vi "BoxExecute.vi"(8 "error in (no error)":errorcluster) -> (0 "error out":errorcluster)   [LabVIEW 2023]
uses:
  BoxStatesEnum.ctl
  BoxNoteState.ctl
  <vilib>/Rock Robotics/WPI/ThirdParty/JAS_Junk/TrajLib/TypeDef/PID_ERROR_TOLERANCE.ctl
  <vilib>/Rock Robotics/WPI/ThirdParty/JAS_Junk/TrajLib/VI/BoolCmd_Recv_Internal.vi
  <vilib>/Rock Robotics/WPI/ThirdParty/JAS_Junk/TrajLib/PIDController_AtSetpoint.vi
  <vilib>/Rock Robotics/WPI/ThirdParty/JAS_Junk/TrajLib/PIDController_SetPIDF.vi
  <vilib>/Rock Robotics/WPI/ThirdParty/JAS_Junk/TrajLib/PIDController_SetDerivativeFilter.vi
  <vilib>/Rock Robotics/WPI/ThirdParty/JAS_Junk/TrajLib/PIDController_SetIntegratorRange.vi
  <vilib>/Rock Robotics/WPI/ThirdParty/JAS_Junk/TrajLib/PIDController_SetTolerancePandV.vi
  <vilib>/Rock Robotics/WPI/ThirdParty/JAS_Junk/TrajLib/PIDController_DisableContinousInput.vi
  <vilib>/Rock Robotics/WPI/ThirdParty/JAS_Junk/TrajLib/PIDController_EnableContinousInput.vi
  <vilib>/Rock Robotics/WPI/ThirdParty/JAS_Junk/TrajLib/PIDController_Reset.vi
  <vilib>/Rock Robotics/WPI/ThirdParty/JAS_Junk/TrajLib/PIDController_New.vi
  <vilib>/Rock Robotics/WPI/ThirdParty/JAS_Junk/TrajLib/PIDController_SetOutputLimits.vi
  <vilib>/Rock Robotics/WPI/ThirdParty/JAS_Junk/TrajLib/VI/PIDController_SetIntegratorZone.vi
  <vilib>/Rock Robotics/WPI/ThirdParty/JAS_Junk/TrajLib/SimpleMotorFF_Calculate.vi
  <vilib>/Rock Robotics/WPI/ThirdParty/JAS_Junk/TrajLib/LinearFilter_ResetToValue.vi
  <vilib>/Rock Robotics/WPI/ThirdParty/JAS_Junk/TrajLib/LinearFilter_Calculate.vi
  <vilib>/Rock Robotics/WPI/ThirdParty/JAS_Junk/TrajLib/SlewRateLimiter_New.vi
  <vilib>/Rock Robotics/WPI/ThirdParty/JAS_Junk/TrajLib/SlewRateLimiter_Reset.vi
  <vilib>/Rock Robotics/WPI/ThirdParty/JAS_Junk/TrajLib/SlewRateLimiter_Calculate.vi
  <vilib>/Rock Robotics/WPI/ThirdParty/JAS_Junk/TrajLib/SlewRateLimiter_SetRate.vi
  <vilib>/Rock Robotics/WPI/ThirdParty/JAS_Junk/TrajLib/VI/BoolCmd_ObtainQueue.vi
  <vilib>/Rock Robotics/WPI/ThirdParty/JAS_Junk/TrajLib/PIDController_NewPeriod.vi
  <vilib>/Rock Robotics/WPI/ThirdParty/JAS_Junk/TrajLib/Util_GetTime.vi
  <vilib>/Rock Robotics/SystemInterfaces/NetworkCommunication/NetComm_UsageReport_report.vi
  <vilib>/Rock Robotics/WPI/ThirdParty/JAS_Junk/TrajLib/VI/Util_GetTime_U32.vi
  BoxGlobals.vi
  BoxNetworkingGlobal.vi
  <vilib>/Utility/semaphor.llb/Obtain Semaphore Reference.vi
  <vilib>/Rock Robotics/WPI/ThirdParty/JAS_Junk/TrajLib/Timer_Reset.vi
  <vilib>/Rock Robotics/WPI/ThirdParty/JAS_Junk/TrajLib/Timer_Start.vi
  <vilib>/Rock Robotics/WPI/ThirdParty/JAS_Junk/TrajLib/Timer_Stop.vi
  <vilib>/Rock Robotics/WPI/ThirdParty/JAS_Junk/TrajLib/LinearFilter_MovingAverage.vi
  <vilib>/Rock Robotics/WPI/ThirdParty/JAS_Junk/TrajLib/LinearFilter_LowPassBW1.vi
  <vilib>/Rock Robotics/WPI/ThirdParty/JAS_Junk/TrajLib/LinearFilter_LowPassBW2.vi
  <vilib>/Rock Robotics/WPI/ThirdParty/JAS_Junk/TrajLib/LinearFilter_HighPassBW1.vi
  <vilib>/Rock Robotics/WPI/ThirdParty/JAS_Junk/TrajLib/LinearFilter_HighPassBW2.vi
  <vilib>/Rock Robotics/SystemInterfaces/Utilities/FPGA_UtilitiesRead LocalTime.vi
  <vilib>/Rock Robotics/WPI/ThirdParty/JAS_Junk/TrajLib/VI/Util_GetTime_U64.vi
  <vilib>/Rock Robotics/WPI/ThirdParty/JAS_Junk/TrajLib/Globals/Util_LibraryGlobals.vi
  <vilib>/Rock Robotics/WPI/ThirdParty/JAS_Junk/TrajLib/PIDController_AdvCalculate_FF_Sp_Pv.vi
  <vilib>/Rock Robotics/WPI/ThirdParty/JAS_Junk/TrajLib/Trajectory_Library.lvlib
panel:
  # "Click here to set min"
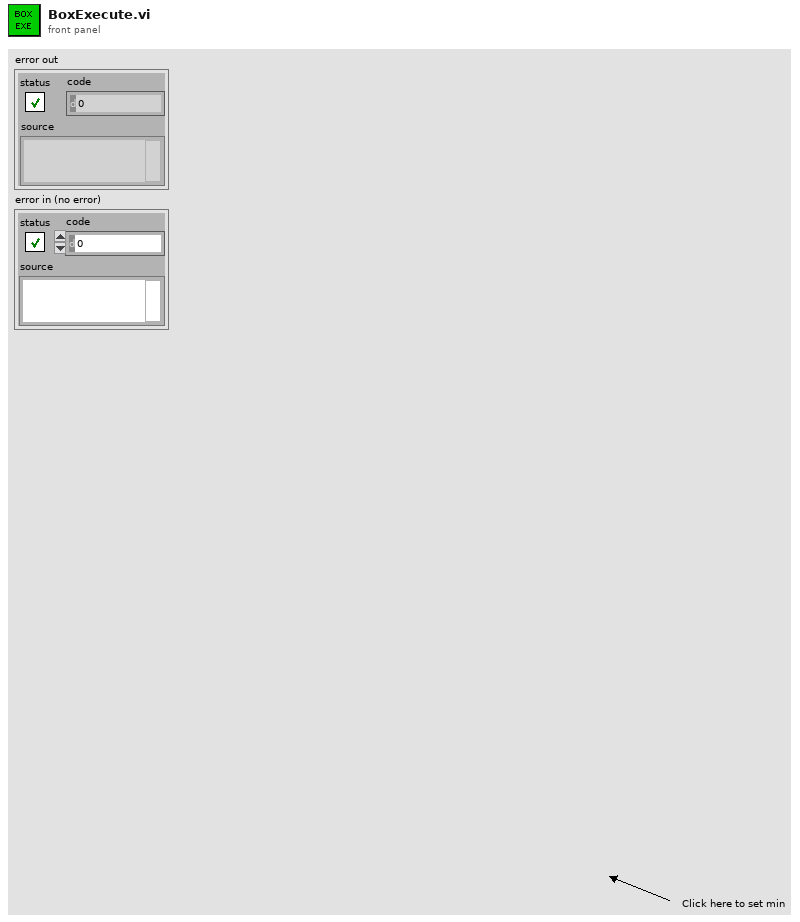
[diagram p1: front panel]
types:
  T1 = typedef "BoxStatesEnum.ctl" = enum16{"get input", "start shoot wheels", "up to speed?", "run intake", "have ring?", "stop intake and shooter", "start intake", "pick up ring or  _ sec?", "stop intake", "start source  intake", "pick up note?", "stop intake shooter", "shoot amp", "used note?", "stop amp intake", "initilization", "pre rev"}
  T2 = typedef "BoxNoteState.ctl" = enum16{"note in shooter wheels", "misaligned note", "no note", "have note"}
  T3 = enum16{"Moving Average", "Low Pass 1st Order Butterworth", "Low Pass 2nd Order Butterworth", "High Pass 1st Order Butterworth", "High Pass 2nd Order Butterworth"}
  T4 = typedef "Trajectory_Library.lvlib/PID_ERROR_TOLERANCE.ctl" = cluster{"PositionTolerance":dbl, "VelocityTolerance":dbl}
  T5 = typedef "WPI_DigitalInputDevRef.ctl" = cluster{"DevStatus":errorcluster, "DIO Channel":T6}
  T6 = typedef "FPGA_DIOChannel.ctl" = enum8{"DIO 0", "DIO 1", "DIO 2", "DIO 3", "DIO 4", "DIO 5", "DIO 6", "DIO 7", "DIO 8", "DIO 9", "DIO MXP 0", "DIO MXP 1", "DIO MXP 2", "DIO MXP 3", "DIO MXP 4", "DIO MXP 5", "DIO MXP 6", "DIO MXP 7", "DIO MXP 8", "DIO MXP 9", "DIO MXP 10", "DIO MXP 11", "DIO MXP 12", "DIO MXP 13", "DIO MXP 14", "DIO MXP 15", "SPI Port CS1", "SPI Port CS2", "SPI Port CS3", "SPI Port MISO", "SPI Port MOSI", "Invalid"}
  T7 = typedef "WPI_MotorControlDeviceRef.ctl" = cluster{"DeviceStatus":errorcluster, "Type":T8, "PWM":cluster{"PWM Channel":T9, "DeadBand":T10}, "CAN":cluster{"Device Number":u8, "SetOutput VI Ref":variant, "GetOutput VI Ref":variant, "Enable VI Ref":variant, "Disable VI Ref":variant, "Data":variant}, "Invert":bool, "DIO PWM":cluster{"PWM \"Enable\" Channel":T9, "DIOChannel":T6, "PWM Rate":dbl}}
  T8 = typedef "WPI_MotorControlType.ctl" = enum16{"PWM", "CAN", "DIO PWM"}
  T9 = typedef "FPGA_DIOPWMChannel.ctl" = enum8{"PWM 0", "PWM 1", "PWM 2", "PWM 3", "PWM 4", "PWM 5", "PWM 6", "PWM 7", "PWM 8", "PWM 9", "PWM MXP 0", "PWM MXP 1", "PWM MXP 2", "PWM MXP 3", "PWM MXP 4", "PWM MXP 5", "PWM MXP 6", "PWM MXP 7", "PWM MXP 8", "PWM MXP 9", "Invalid"}
  T10 = typedef "WPI_PWMDeadband.ctl" = cluster{"Name":string, "maxPositivePwm":i32, "minPositivePwm":i32, "centerPwm":i32, "maxNegativePwm":i32, "minNegativePwm":i32, "angularRange":u16}
  T11 = typedef "Trajectory_Library.lvlib/TIMER.ctl" = cluster{"StartTime":dbl, "Accumulated TIme":dbl, "Running":bool, "semaphore":T12}
  T12 = typedef "Semaphore RefNum" = refnum<k1>
  T13 = typedef "Trajectory_Library.lvlib/SIMPLE_MOTOR_FF.ctl" = cluster{"Ks":dbl, "Kv":dbl, "Ka":dbl, "KnInv":dbl}
  T14 = typedef "Trajectory_Library.lvlib/PID_ADV_LIMITS.ctl" = cluster{"MaxInput":dbl, "MinInput":dbl, "Continuous":bool, "MaxOutput":dbl, "MinOutput":dbl}
  T15 = typedef "Trajectory_Library.lvlib/PID_ADV_TUNING.ctl" = cluster{"Kf":dbl, "Kp":dbl, "Ki":dbl, "Kd":dbl, "MaximumIntegral":dbl, "MinimumIntegral":dbl, "Filter Derivative":bool, "IntegralZone":dbl}
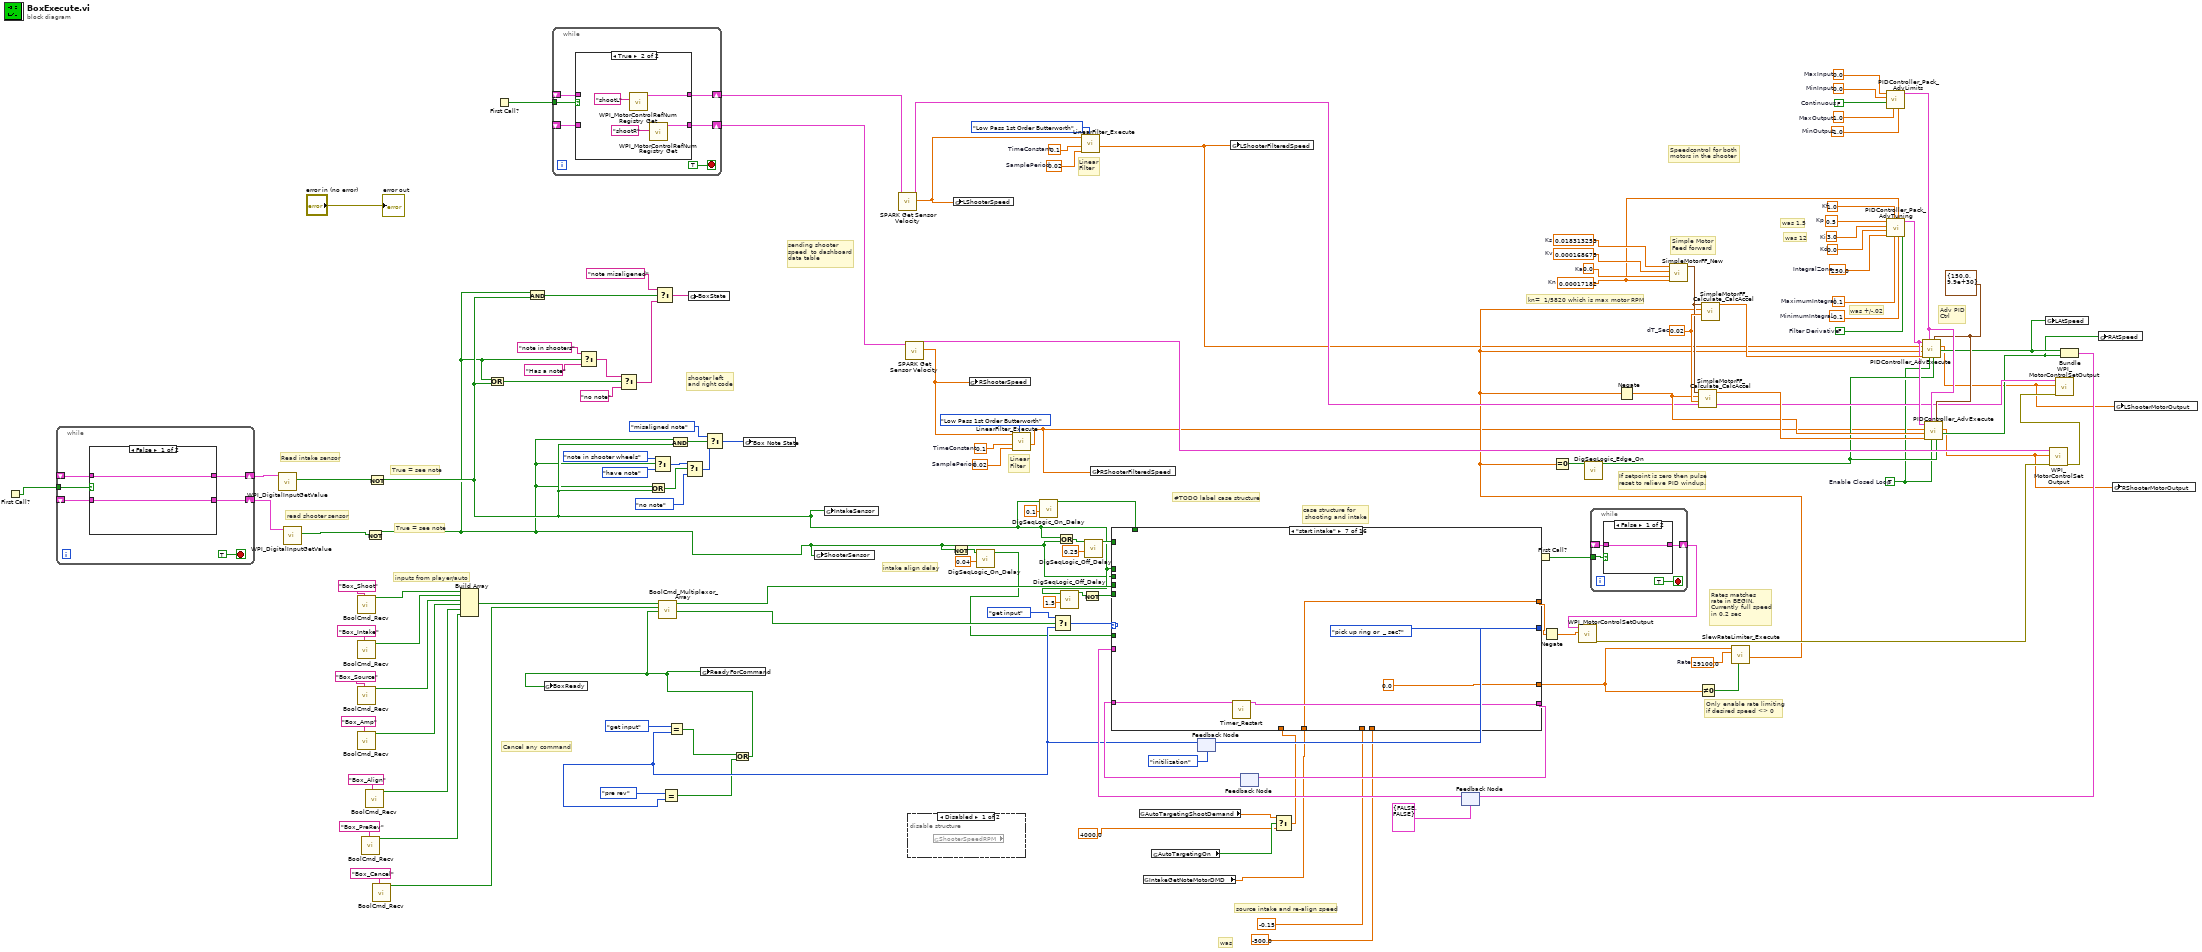
[diagram p0: block diagram]
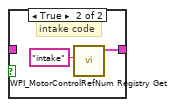
[diagram p3: hidden frame]
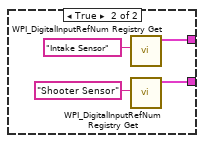
[diagram p4: hidden frame]
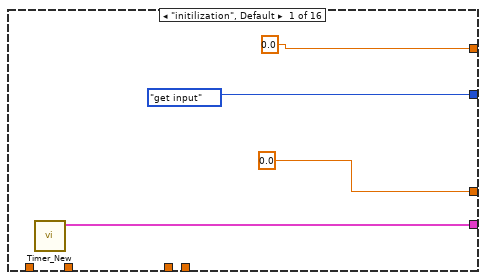
[diagram p6: hidden frame]
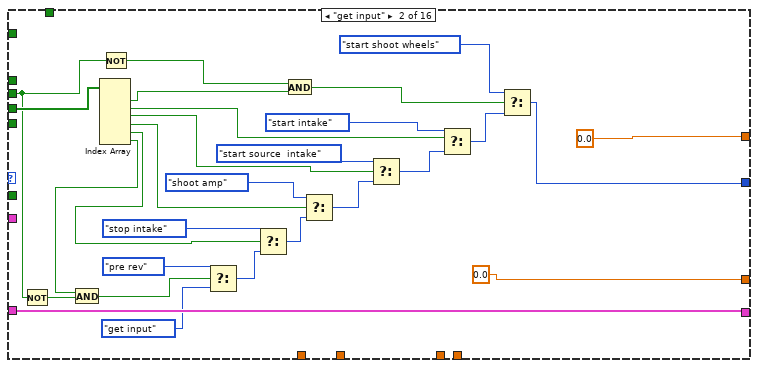
[diagram p7: hidden frame]
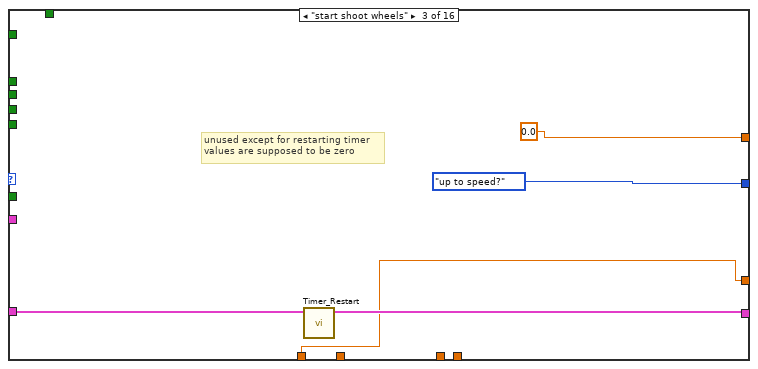
[diagram p8: hidden frame]
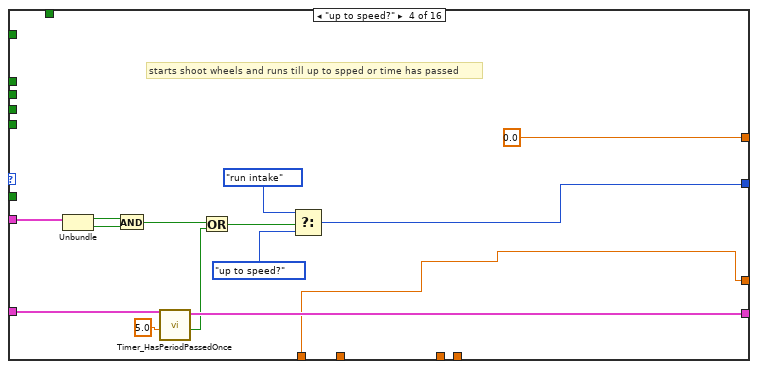
[diagram p9: hidden frame]
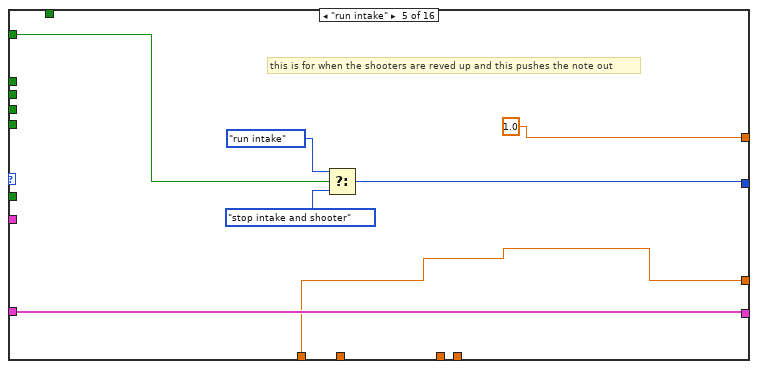
[diagram p10: hidden frame]
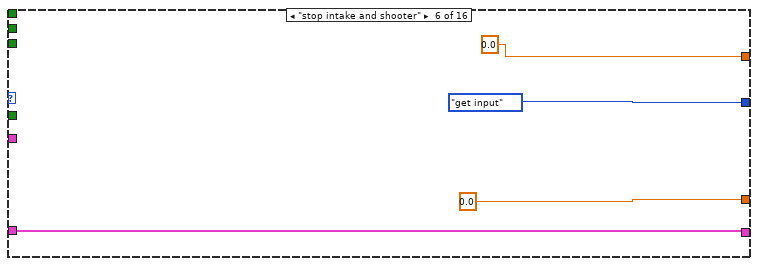
[diagram p11: hidden frame]
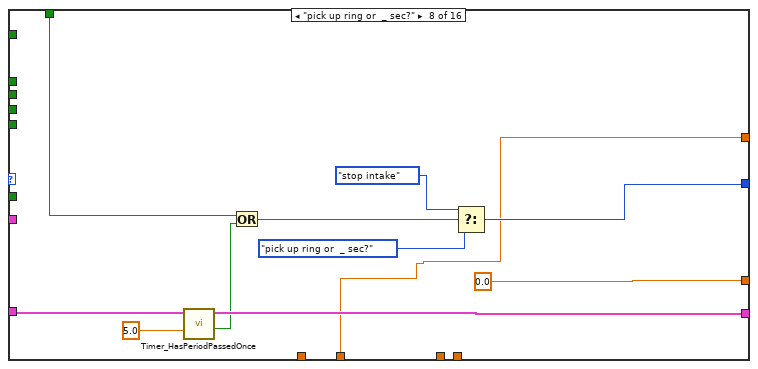
[diagram p12: hidden frame]
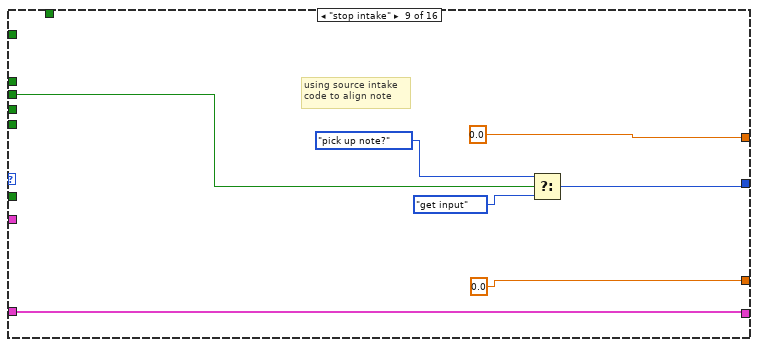
[diagram p13: hidden frame]
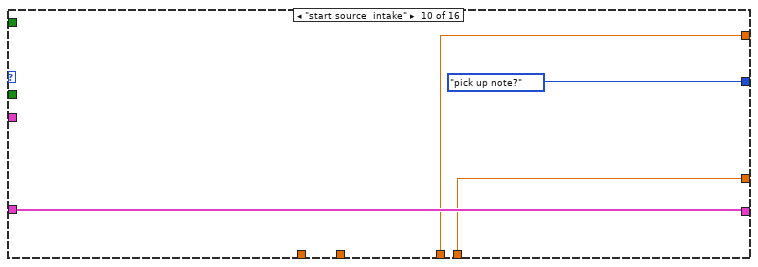
[diagram p14: hidden frame]
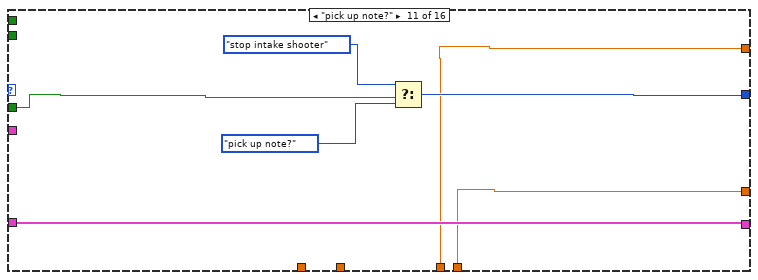
[diagram p15: hidden frame]
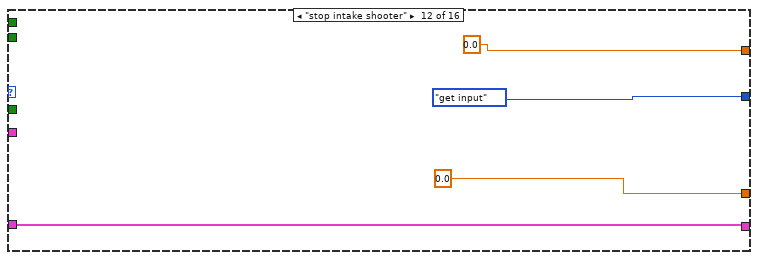
[diagram p16: hidden frame]
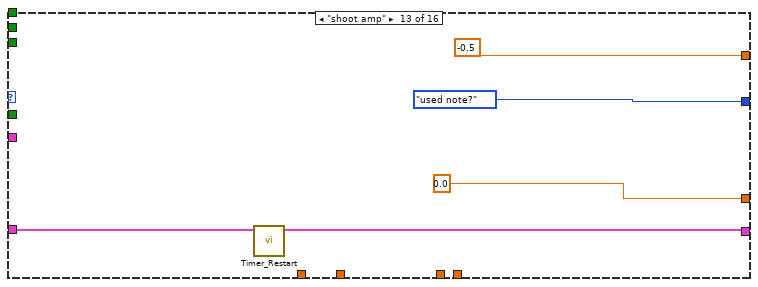
[diagram p17: hidden frame]
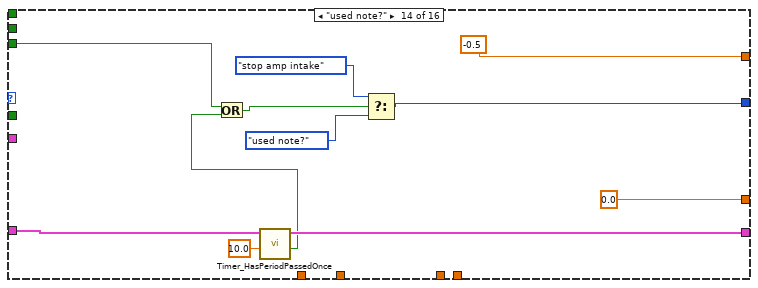
[diagram p18: hidden frame]
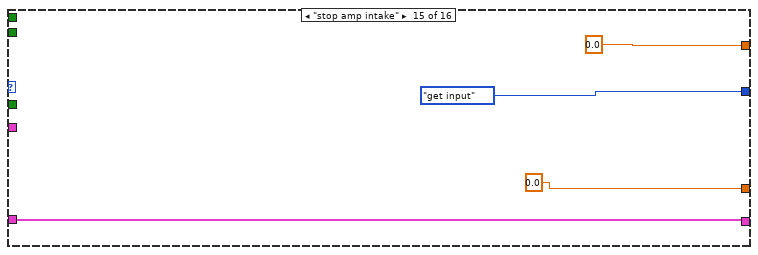
[diagram p19: hidden frame]
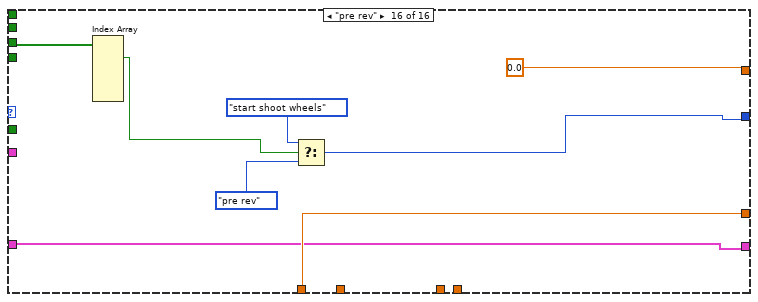
[diagram p20: hidden frame]
diagram:
  w6 = 250.0  # IntegralZone
  w41 = 29100.0  # Rate
  w79 = 0.02  # SamplePeriod
  w78 = 0.1  # TimeConstant
  w83 = 0.02  # SamplePeriod
  w82 = 0.1  # TimeConstant
  w38 = TRUE  # Enable Closed Loop
  w87 = T4 {"PositionTolerance"=150.0, "VelocityTolerance"=9.9e+30} ("PID Error Tolerance")
  w99 = 0.00017182  # Kn
  w102 = 0.018313253  # Ks
  w101 = 0.000168675  # Kv
  w100 = 0.0  # Ka
  w97 = 0.5  # Kp
  w96 = 3.0  # Ki
  w95 = 0.0  # Kd
  w98 = 1.0  # Kf
  w94 = 0.1  # MaximumIntegral
  w93 = -0.1  # MinimumIntegral
  w92 = FALSE  # Filter Derivative
  w106 = 0.0  # MinInput
  w105 = FALSE  # Continuous
  w104 = 1.0  # MaxOutput
  w103 = -1.0  # MinOutput
  w107 = 0.0  # MaxInput
  w91 = 0.02  # dT_Sec
  # "intake align delay"
  # "was"
  # "source intake and re-align speed"
  # "was 12"
  # "was 1.5"
  # "True = see note"
  # "True = see note"
  # "read shooter sensor"
  # "Read intake sensor"
  # "was +/-.02"
  # "If setpoint is zero then pulse\nreset to relieve PID windup."
  # "Rates matches\nrate in BEGIN.  \nCurrently full speed\nin 0.2 sec"
  # "Only enable rate limiting\nif desired speed <> 0"
  # "#TODO label case structure"
  # "inputs from player/auto"
  # "Linear\nFilter"
  # "Linear\nFilter"
  # "Speedcontrol for both \nmotors in the shooter"
  # "Simple Motor\nFeed forward"
  # "Adv PID\nCtrl"
  # "Cancel any command"
  # "kn=  1/5820 which is max motor RPM"
  # "case structure for\n shooting and intake"
  # "sending shooter \nspeed  to dashboard \ndata table"
  # "shooter left \nand right code"
  n1 = First Call?() -> (First Call?: T/F=w36:bool)
  n2 = while {
    tunnel: w36 -> [w137]
    shift-right: [w138] -> w111
    shift-left: _ -> [w136]
    shift-right: [w139] -> w112
    shift-left: _ -> [w135]
    stop <- TRUE stop-if-true
    n3 = case shown="False" w137 {
      tunnel: [w140 w145] -> w139
      tunnel: [w141 w144] -> w138
      tunnel: w136 -> [w141 _]
      tunnel: w135 -> [w140 _]
      frame False {
      }
      frame True {
        n4 = call <vilib>:"WPI_DigitalInputRefNum Registry Get.vi"("refnum name"="Intake Sensor") -> ("DigitalInputDevRef"=w144:T5)  [unwired: 9 in, 1 out]
        n5 = call <vilib>:"WPI_DigitalInputRefNum Registry Get.vi"("refnum name"="Shooter Sensor") -> ("DigitalInputDevRef"=w145:T5)  [unwired: 9 in, 1 out]
      }
    }
  }
  n6 = call <vilib>:"WPI_DigitalInputGetValue.vi"("DigitalInputDevRef"=w111) -> ("Value"=w66:bool)  [unwired: 8 in, 2 out]
  n7 = call <vilib>:"WPI_DigitalInputGetValue.vi"("DigitalInputDevRef"=w112) -> ("Value"=w65:bool)  [unwired: 8 in, 2 out]
  n8 = call <vilib>:"BoolCmd_Recv.vi"("Command Name"="Box_Shoot") -> ("New Request"=w122:bool)  [unwired: 9 in, 1 out]
  n9 = call <vilib>:"BoolCmd_Recv.vi"("Command Name"="Box_Intake") -> ("New Request"=w123:bool)  [unwired: 9 in, 1 out]
  n10 = call <vilib>:"BoolCmd_Recv.vi"("Command Name"="Box_Source") -> ("New Request"=w126:bool)  [unwired: 9 in, 1 out]
  n11 = call <vilib>:"BoolCmd_Recv.vi"("Command Name"="Box_Amp") -> ("New Request"=w127:bool)  [unwired: 9 in, 1 out]
  n12 = call <vilib>:"BoolCmd_Recv.vi"("Command Name"="Box_PreRev") -> ("New Request"=w27:bool)  [unwired: 9 in, 1 out]
  n13 = call <vilib>:"BoolCmd_Recv.vi"("Command Name"="Box_Align") -> ("New Request"=w44:bool)  [unwired: 9 in, 1 out]
  n14 = Not(x=w65) -> (.not. x?=w3:bool)
  n15 = Not(x=w66) -> (.not. x?=w15:bool)
  n16 = call <vilib>:"BoolCmd_Recv.vi"("Command Name"="Box_Cancel") -> ("New Request"=w120:bool)  [unwired: 9 in, 1 out]
  n17 = Build Array(w122, w123, w126, w127, w44, w27) -> (w121:bool[])
  n18 = Or(x=w3, y=w15) -> (x .or. y?=w73:bool)
  n19 = First Call?() -> (First Call?: T/F=w37:bool)
  n20 = And(x=w3, y=w15) -> (x .and. y?=w74:bool)
  n21 = while {
    tunnel: w37 -> [w149]
    shift-right: [w151] -> w133
    shift-left: _ -> [w147]
    shift-right: [w150] -> w132
    shift-left: _ -> [w146]
    stop <- TRUE stop-if-true
    n22 = case shown="True" w149 {
      tunnel: [w153 w155] -> w151
      tunnel: [w152 w154] -> w150
      tunnel: w147 -> [w153 _]
      tunnel: w146 -> [w152 _]
      frame False {
      }
      frame True {
        n23 = call <vilib>:"WPI_MotorControlRefNum Registry Get.vi"("refnum name"="shootL") -> ("MotorControlDevRef"=w155:T7)  [unwired: 9 in, 1 out]
        n24 = call <vilib>:"WPI_MotorControlRefNum Registry Get.vi"("refnum name"="shootR") -> ("MotorControlDevRef"=w154:T7)  [unwired: 9 in, 1 out]
      }
    }
  }
  n25 = Select(t="note in shooters", s=w3, f="Has a note") -> (s? t:f=w72:string)
  n26 = Select(t=w72, s=w73, f="no note") -> (s? t:f=w70:string)
  n27 = Or(x=w3, y=w15) -> (x .or. y?=w63:bool)
  n28 = Select(t=BoxNoteState."note in shooter wheels" ("Box Note State"), s=w3, f=BoxNoteState."have note" ("Box Note State")) -> (s? t:f=w62:T2)
  n29 = Select(t="note misaligened", s=w74, f=w70) -> (s? t:f=w14:string)
  n30 = And(x=w3, y=w15) -> (x .and. y?=w64:bool)
  n31 = Select(t=w62, s=w63, f=BoxNoteState."no note" ("Box Note State")) -> (s? t:f=w61:T2)
  n32 = global write "BoxNetworkingGlobal.vi" "BoxState"(w14) -> ()
  n33 = Select(t=BoxNoteState."misaligned note" ("Box Note State"), s=w64, f=w61) -> (s? t:f=w56:T2)
  n34 = global write "BoxGlobals.vi" "Box Note State"(w56) -> ()
  n35 = global write "BoxNetworkingGlobal.vi" "ShooterSensor"(w3) -> ()
  n36 = global write "BoxNetworkingGlobal.vi" "IntakeSensor"(w15) -> ()
  n37 = call <vilib>:"SPARK Get Sensor Velocity.vi"("MotorControlDevRef in"=w133) -> ("Sensor Velocity"=w23:dbl, "MotorControlDevRef out"=w80:T7)  [unwired: 7 in, 2 out]
  n38 = call <vilib>:"SPARK Get Sensor Velocity.vi"("MotorControlDevRef in"=w132) -> ("Sensor Velocity"=w21:dbl, "MotorControlDevRef out"=w55:T7)  [unwired: 7 in, 2 out]
  n39 = disable-structure shown="Disabled" {
    frame Disabled {
      n40 = global read "BoxGlobals.vi" "ShooterSpeedRPM"() -> ()  [unwired: 1 out]
    }
    frame Enabled {
    }
  }
  n41 = Not(x=w3) -> (.not. x?=w5:bool)
  n42 = global write "BoxNetworkingGlobal.vi" "LShooterSpeed"(w23) -> ()
  n43 = global write "BoxNetworkingGlobal.vi" "RShooterSpeed"(w21) -> ()
  n44 = call <vilib>:"DigSeqLogic_On_Delay.vi"("Delay"=0.04, "Input"=w5) -> ("Output"=w2:bool)  [unwired: 8 in, 1 out]
  n45 = call <vilib>:"LinearFilter_Execute.vi"("Filter Type"=T3."Low Pass 1st Order Butterworth", "SamplePeriod"=w83, "TimeConstant"=w82, "Input"=w21) -> ("Output"=w20:dbl)  [unwired: 6 in, 1 out]
  n46 = call <vilib>:"DigSeqLogic_On_Delay.vi"("Delay"=0.1 ("On Delay Time\nSeconds"), "Input"=w15) -> ("Output"=w29:bool)  [unwired: 8 in, 1 out]
  n47 = Or(x=w15, y=w3) -> (x .or. y?=w50:bool)
  n48 = call <vilib>:"DigSeqLogic_Off_Delay.vi"("Delay"=1.5 ("Off Delay Tme\nSeconds"), "Input"=w15) -> ("Output"=w47:bool)  [unwired: 8 in, 1 out]
  n49 = call <vilib>:"LinearFilter_Execute.vi"("Filter Type"=T3."Low Pass 1st Order Butterworth", "SamplePeriod"=w79, "TimeConstant"=w78, "Input"=w23) -> ("Output"=w22:dbl)  [unwired: 6 in, 1 out]
  n50 = Not(x=w47) -> (.not. x?=w46:bool)
  n51 = call <vilib>:"DigSeqLogic_Off_Delay.vi"("Delay"=0.25 ("Off Delay Tme\nSeconds"), "Input"=w50) -> ("Output"=w49:bool)  [unwired: 8 in, 1 out]
  n52 = global write "BoxNetworkingGlobal.vi" "RShooterFilteredSpeed"(w20) -> ()
  n53 = global read "BoxGlobals.vi" "AutoTargetingShootDemand"() -> (w26:dbl)
  n54 = global read "BoxGlobals.vi" "IntakeGetNoteMotorDMD"() -> (w32:dbl)
  n55 = global read "BoxGlobals.vi" "AutoTargetingOn"() -> (w25:bool)
  n56 = feedback #1(BoxStatesEnum."initilization") -> (w10:T1)
  n57 = Equal?(x=BoxStatesEnum."pre rev" ("Box states"), y=w10) -> (x = y?=w9:bool)
  n58 = Equal?(x=BoxStatesEnum."get input" ("Box states"), y=w10) -> (x = y?=w8:bool)
  n59 = Or(x=w8, y=w9) -> (x .or. y?=w7:bool)
  n60 = global write "BoxNetworkingGlobal.vi" "BoxReady"(w7) -> ()
  n61 = call <vilib>:"BoolCmd_Multiplexor_Array.vi"("Ready"=w7, "Command Cancel"=w120, "Commands"=w121) -> ("Do Cancel"=w114:bool, "Do Command"=w116:bool[])  [unwired: 7 in]
  n62 = global write "BoxGlobals.vi" "ReadyForCommand"(w7) -> ()
  n63 = Select(t=BoxStatesEnum."get input" ("Box states"), s=w114, f=w10) -> (s? t:f=w115:T1)
  n64 = global write "BoxNetworkingGlobal.vi" "LShooterFilteredSpeed"(w22) -> ()
  n65 = feedback #2() -> (w75:T11)  [unwired: 1 in]
  n66 = Select(t=w26, s=w25, f=4000.0) -> (s? t:f=w24:dbl)
  n67 = feedback #3(cluster{bool, bool} {FALSE, FALSE}) -> (w129:cluster{bool, bool})
  n68 = case shown="\"start intake\"" w115 {
    tunnel: [BoxStatesEnum."get input" ("Box states") w183 BoxStatesEnum."up to speed?" ("Box states") w203 w212 BoxStatesEnum."get input" ("Box states") BoxStatesEnum."pick up ring or  _ sec?" ("Box states") w232 w239 BoxStatesEnum."pick up note?" ("Box states") w250 BoxStatesEnum."get input" ("Box states") BoxStatesEnum."used note?" ("Box states") w269 BoxStatesEnum."get input" ("Box states") w282] -> w130
    tunnel: w129 -> [_ _ _ w206 _ _ _ _ _ _ _ _ _ _ _ _]
    tunnel: [0.0 0.0 w190 w195 w209 0.0 0.0 0.0 0.0 w243 w248 0.0 0.0 0.0 0.0 w283] -> w39
    tunnel: [0.0 0.0 0.0 0.0 1.0 0.0 w220 w226 0.0 w244 w249 0.0 -0.5 -0.5 0.0 0.0] -> w52
    tunnel: w116 -> [_ w188 _ _ _ _ _ _ _ _ _ _ _ _ _ w280]
    tunnel: w15 -> [_ _ _ _ _ _ _ _ _ _ _ _ _ _ _ _]
    tunnel: w3 -> [_ w165 _ _ _ _ _ _ w236 _ _ _ _ _ _ _]
    tunnel: [w158 w175 w191 w200 w211 w216 w222 w228 w240 w245 w253 w254 w258 w267 w274 w281] -> w76
    tunnel: w75 -> [_ w175 w192 w201 w211 w216 w221 w230 w240 w245 w253 w254 w259 w268 w274 w281]
    tunnel: w49 -> [_ _ _ _ w210 _ _ _ _ _ _ _ _ _ _ _]
    tunnel: w46 -> [_ _ _ _ _ _ _ _ _ _ _ _ _ w263 _ _]
    tunnel: w24 -> [_ _ w190 w195 w209 _ _ _ _ _ _ _ _ _ _ w283]
    tunnel: w32 -> [_ _ _ _ _ _ w220 w226 _ _ _ _ _ _ _ _]
    tunnel: w29 -> [_ _ _ _ _ _ _ w225 _ _ _ _ _ _ _ _]
    tunnel: -0.15 -> [_ _ _ _ _ _ _ _ _ w244 w249 _ _ _ _ _]
    tunnel: -500.0 -> [_ _ _ _ _ _ _ _ _ w243 w248 _ _ _ _ _]
    tunnel: w2 -> [_ _ _ _ _ _ _ _ _ _ w247 _ _ _ _ _]
    frame "initilization", Default {
      n69 = call <vilib>:"Timer_New.vi"() -> ("TIMER"=w158:T11)  [unwired: 11 in]
    }
    frame "get input" {
      n70 = Not(x=w165) -> (.not. x?=w163:bool)
      n71 = Index Array(array=w188) -> (element #1=w173:bool, element #2=w180:bool, element #3=w179:bool, element #4=w178:bool, element #5=w169:bool, element #6=w164:bool)  [unwired: 6 in]
      n72 = And(x=w164, y=w163) -> (x .and. y?=w162:bool)
      n73 = Not(x=w165) -> (.not. x?=w172:bool)
      n74 = Select(t=BoxStatesEnum."pre rev" ("Box states"), s=w162, f=BoxStatesEnum."get input" ("Box states")) -> (s? t:f=w168:T1)
      n75 = Select(t=BoxStatesEnum."stop intake" ("Box states"), s=w169, f=w168) -> (s? t:f=w171:T1)
      n76 = And(x=w172, y=w173) -> (x .and. y?=w174:bool)
      n77 = Select(t=BoxStatesEnum."shoot amp" ("Box states"), s=w178, f=w171) -> (s? t:f=w184:T1)
      n78 = Select(t=BoxStatesEnum."start source  intake", s=w179, f=w184) -> (s? t:f=w185:T1)
      n79 = Select(t=BoxStatesEnum."start intake" ("Box states"), s=w180, f=w185) -> (s? t:f=w186:T1)
      n80 = Select(t=BoxStatesEnum."start shoot wheels" ("Box states"), s=w174, f=w186) -> (s? t:f=w183:T1)
    }
    frame "start shoot wheels" {
      # "unused except for restarting timer\nvalues are supposed to be zero"
      n81 = call <vilib>:"Timer_Restart.vi"("in Timer"=w192) -> ("out Timer"=w191:T11)  [unwired: 10 in]
    }
    frame "up to speed?" {
      # "starts shoot wheels and runs till up to spped or time has passed"
      n82 = Unbundle(w206) -> (w205:bool, w204:bool)
      n83 = And(x=w205, y=w204) -> (x .and. y?=w198:bool)
      n84 = call <vilib>:"Timer_HasPeriodPassedOnce.vi"("Period"=5.0, "in Timer"=w201) -> ("Expired"=w196:bool, "out Timer"=w200:T11)  [unwired: 7 in, 1 out]
      n85 = Or(x=w198, y=w196) -> (x .or. y?=w197:bool)
      n86 = Select(t=BoxStatesEnum."run intake" ("Box states"), s=w197, f=BoxStatesEnum."up to speed?" ("Box states")) -> (s? t:f=w203:T1)
    }
    frame "run intake" {
      # "this is for when the shooters are reved up and this pushes the note out"
      n87 = Select(t=BoxStatesEnum."run intake" ("Box states"), s=w210, f=BoxStatesEnum."stop intake and shooter" ("Box states")) -> (s? t:f=w212:T1)
    }
    frame "stop intake and shooter" {
    }
    frame "start intake" {
      n88 = call <vilib>:"Timer_Restart.vi"("in Timer"=w221) -> ("out Timer"=w222:T11)  [unwired: 10 in]
    }
    frame "pick up ring or  _ sec?" {
      n89 = call <vilib>:"Timer_HasPeriodPassedOnce.vi"("Period"=5.0, "in Timer"=w230) -> ("Expired"=w227:bool, "out Timer"=w228:T11)  [unwired: 7 in, 1 out]
      n90 = Or(x=w225, y=w227) -> (x .or. y?=w231:bool)
      n91 = Select(t=BoxStatesEnum."stop intake" ("Box states"), s=w231, f=BoxStatesEnum."pick up ring or  _ sec?" ("Box states")) -> (s? t:f=w232:T1)
    }
    frame "stop intake" {
      # "using source intake \ncode to align note"
      n92 = Select(t=BoxStatesEnum."pick up note?" ("Box states"), s=w236, f=BoxStatesEnum."get input" ("Box states")) -> (s? t:f=w239:T1)
    }
    frame "start source  intake" {
    }
    frame "pick up note?" {
      n93 = Select(t=BoxStatesEnum."stop intake shooter" ("Box states"), s=w247, f=BoxStatesEnum."pick up note?" ("Box states")) -> (s? t:f=w250:T1)
    }
    frame "stop intake shooter" {
    }
    frame "shoot amp" {
      n94 = call <vilib>:"Timer_Restart.vi"("in Timer"=w259) -> ("out Timer"=w258:T11)  [unwired: 10 in]
    }
    frame "used note?" {
      n95 = call <vilib>:"Timer_HasPeriodPassedOnce.vi"("Period"=10.0, "in Timer"=w268) -> ("Expired"=w265:bool, "out Timer"=w267:T11)  [unwired: 7 in, 1 out]
      n96 = Or(x=w263, y=w265) -> (x .or. y?=w264:bool)
      n97 = Select(t=BoxStatesEnum."stop amp intake" ("Box states"), s=w264, f=BoxStatesEnum."used note?" ("Box states")) -> (s? t:f=w269:T1)
    }
    frame "stop amp intake" {
    }
    frame "pre rev" {
      n98 = Index Array(array=w280) -> (element #1=w278:bool)  [unwired: 6 in, 5 out]
      n99 = Select(t=BoxStatesEnum."start shoot wheels" ("Box states"), s=w278, f=BoxStatesEnum."pre rev" ("Box states")) -> (s? t:f=w282:T1)
    }
  }
  n100 = feedback-in #1(w130) -> ()
  n101 = feedback-in #2(w76) -> ()
  n102 = First Call?() -> (First Call?: T/F=w35:bool)
  n103 = Negate(x=w52) -> (-x=w53:dbl)
  n104 = while {
    tunnel: w35 -> [w288]
    shift-right: [w289] -> w128
    shift-left: _ -> [w286]
    stop <- TRUE stop-if-true
    n105 = case shown="False" w288 {
      tunnel: [w290 w291] -> w289
      tunnel: w286 -> [w290 _]
      frame False {
      }
      frame True {
        # "intake code"
        n106 = call <vilib>:"WPI_MotorControlRefNum Registry Get.vi"("refnum name"="intake") -> ("MotorControlDevRef"=w291:T7)  [unwired: 9 in, 1 out]
      }
    }
  }
  n107 = call <vilib>:"WPI_MotorControlSetOutput.vi"("Output"=w53, "MotorControlDevRef"=w128) -> ("error out"=w34:errorcluster)  [unwired: 7 in, 2 out]
  n108 = call <vilib>:"SimpleMotorFF_New.vi"("Kn"=w99, "Ka"=w100, "Kv"=w101, "Ks"=w102) -> ("SIMPLE_MOTOR_FF"=w90:T13)  [unwired: 7 in]
  n109 = Not Equal To 0?(x=w39) -> (x != 0?=w40:bool)
  n110 = call <vilib>:"SlewRateLimiter_Execute.vi"("Enable"=w40, "PositiveRate"=w41, "Input"=w39) -> ("Output"=w31:dbl)  [unwired: 7 in, 1 out]
  n111 = Equal To 0?(x=w31) -> (x = 0?=w43:bool)
  n112 = call <vilib>:"DigSeqLogic_Edge_On.vi"("Input"=w43) -> ("On Edge"=w42:bool)  [unwired: 10 in]
  n113 = Negate(x=w31) -> (-x=w84:dbl)
  n114 = call <vilib>:"SimpleMotorFF_Calculate_CalcAccel.vi"("dT_Sec"=w91, "VelSp"=w84, "SIMPLE_MOTOR_FF"=w90) -> ("FeedForward"=w86:dbl)  [unwired: 8 in]
  n115 = call <vilib>:"SimpleMotorFF_Calculate_CalcAccel.vi"("dT_Sec"=w91, "VelSp"=w31, "SIMPLE_MOTOR_FF"=w90) -> ("FeedForward"=w108:dbl)  [unwired: 8 in]
  n116 = call <vilib>:"PIDController_Pack_AdvLimits.vi"("MinOutput"=w103, "MaxOutput"=w104, "Continuous"=w105, "MinInput"=w106, "MaxInput"=w107) -> ("Adv PID Limits"=w88:T14)  [unwired: 6 in]
  n117 = call <vilib>:"PIDController_Pack_AdvTuning.vi"("Filter Derivative"=w92, "MinimumIntegral"=w93, "Kn"=w99, "MaximumIntegral"=w94, "Kf"=w98, "IntegralZone"=w6, "Kd"=w95, "Ki"=w96, "Kp"=w97) -> ("Adv PID Tuning"=w89:T15)  [unwired: 2 in]
  n118 = call <vilib>:"PIDController_AdvExecute.vi"("Reset"=w42, "PID Error Tolerance"=w87, "Auto"=w38, "Adv PID Limits"=w88, "FF-FeedForward"=w108, "SP-SetPoint"=w31, "PV-Measurement"=w22, "Adv PID Tuning"=w89) -> ("AtSetpoint"=w19:bool, "CO-ControlOutput"=w17:dbl)  [unwired: 1 in, 1 out]
  n119 = call <vilib>:"PIDController_AdvExecute.vi"("Reset"=w42, "PID Error Tolerance"=w87, "Auto"=w38, "Adv PID Limits"=w88, "FF-FeedForward"=w86, "SP-SetPoint"=w84, "PV-Measurement"=w20, "Adv PID Tuning"=w89) -> ("AtSetpoint"=w18:bool, "CO-ControlOutput"=w16:dbl)  [unwired: 1 in, 1 out]
  n120 = global write "BoxNetworkingGlobal.vi" "LAtSpeed"(w19) -> ()
  n121 = call <vilib>:"WPI_MotorControlSetOutput.vi"("error in (no error)"=w34, "Output"=w16, "MotorControlDevRef"=w55) -> ("error out"=w33:errorcluster)  [unwired: 6 in, 2 out]
  n122 = call <vilib>:"WPI_MotorControlSetOutput.vi"("error in (no error)"=w33, "Output"=w17, "MotorControlDevRef"=w80) -> ()  [unwired: 6 in, 3 out]
  n123 = Bundle("AtSetpoint"=w19, "AtSetpoint"=w18) -> (w85:cluster{"AtSetpoint":bool, "AtSetpoint":bool})  [unwired: 1 in]
  n124 = feedback-in #3(w85) -> ()
  n125 = global write "BoxNetworkingGlobal.vi" "RAtSpeed"(w18) -> ()
  n126 = global write "BoxNetworkingGlobal.vi" "RShooterMotorOutput"(w16) -> ()
  n127 = global write "BoxNetworkingGlobal.vi" "LShooterMotorOutput"(w17) -> ()
  "error out" <- "error in (no error)"
